vi "In.vi"(8 "error in (no error)":errorcluster, 11 "FlipMir in":refnum<class "FlipMir.lvclass">) -> (0 "error out":errorcluster, 3 "FlipMir out":refnum<class "FlipMir.lvclass">)   [LabVIEW 2016, in "FlipMir.lvclass"]
uses:
  FlipMir.lvclass
  FlipMir.lvclass/FlipMir.ctl
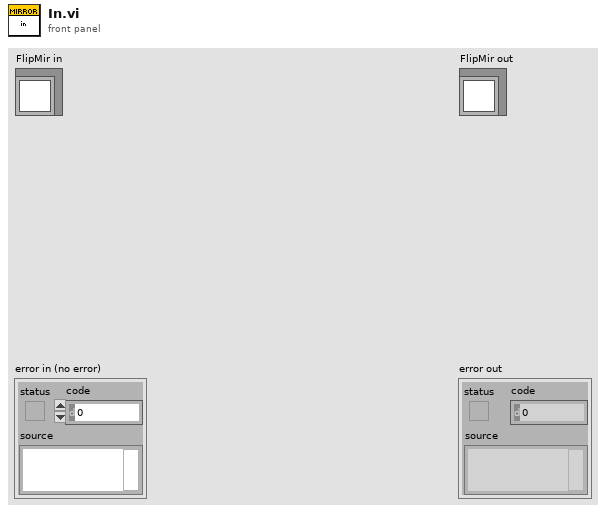
[diagram p1: front panel]
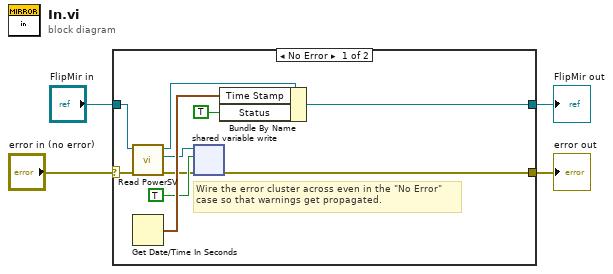
[diagram p0: block diagram]
diagram:
  n1 = case shown="No Error" "error in (no error)" {
    selector: "error in (no error)" -> [w5 w16]
    tunnel: [w6 w16] -> w3
    tunnel: [w14 w15] -> w1
    tunnel: "FlipMir in" -> [w10 w15]
    frame No Error {
      # "Wire the error cluster across even in the \"No Error\"\ncase so that warnings get propagated."
      n2 = call-dynamic "Read PowerSV.vi"("error in (no error)"=w5, "FlipMir in"=w10) -> ("error out"=w7:errorcluster, "PowerSV"=w8:refnum<k21>, "FlipMir out"=w9:refnum<class "FlipMir.lvclass">)  [unwired: 7 in]
      n3 = Get Date/Time In Seconds() -> (seconds since 1Jan1904=w13:timestamp)
      n4 = shared-variable-write(w8, w7, TRUE ("data in")) -> (w6:errorcluster)  [unwired: 1 out]
      n5 = Bundle By Name(cluster=w9, "Time Stamp"=w13, "Status"=TRUE) -> (w14:refnum<class "FlipMir.lvclass">)
    }
    frame Error {
    }
  }
  "error out" <- w3
  "FlipMir out" <- w1
